vi "Write Element of Seq_GUI.vi"(8 "error in (no error)":errorcluster, 9 "GUI_Handler_Seq.lvclass":refnum<class "GUI_Handler_Seq.lvclass">, 10 "index":i32, 11 "GUI_Handler_Main in":refnum<class "GUI_Handler_Main.lvclass">) -> (0 "error out":errorcluster, 3 "GUI_Handler_Main out":refnum<class "GUI_Handler_Main.lvclass">)   [LabVIEW 2019, in "GUI_Handler_Main.lvclass"]
uses:
  GUI_Handler_Main.lvclass
  GUIHandler/GUI_Handler_Seq.lvclass
  GUI_Handler_Main.lvclass/GUI_Handler_Main.ctl
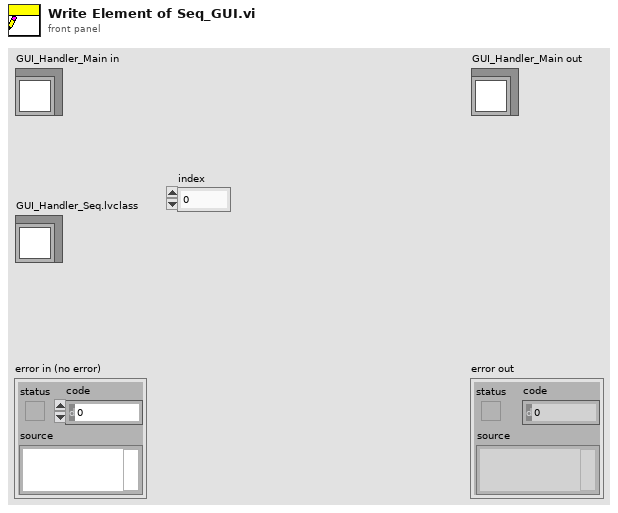
[diagram p1: front panel]
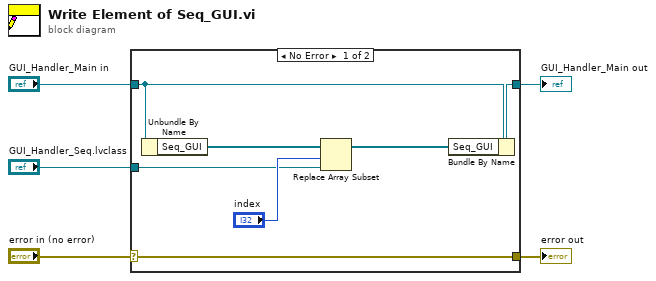
[diagram p0: block diagram]
diagram:
  n1 = case shown="No Error" "error in (no error)" {
    selector: "error in (no error)" -> [w12 w13]
    tunnel: [w12 w13] -> w4
    tunnel: [w11 w14] -> w2
    tunnel: "GUI_Handler_Main in" -> [w10 w14]
    tunnel: "GUI_Handler_Seq.lvclass" -> [w6 _]
    frame No Error {
      n2 = Unbundle By Name(w10) -> ("Seq_GUI"=w9:refnum<class "GUI_Handler_Seq.lvclass">[])
      n3 = Replace Array Subset(array=w9, new element=w6, index="index") -> (w8:refnum<class "GUI_Handler_Seq.lvclass">[])
      n4 = Bundle By Name(cluster=w10, "Seq_GUI"=w8) -> (w11:refnum<class "GUI_Handler_Main.lvclass">)
    }
    frame Error {
    }
  }
  "error out" <- w4
  "GUI_Handler_Main out" <- w2
